vi "PH_ImageOperator.get COG.vi"(1 "Image":T1, 5 "error in (no error)":errorcluster) -> (16 "CoG-x":sgl, 17 "CoG-y":sgl, 19 "error out":errorcluster)   [LabVIEW 2014, in "PH_ImageOperator.lvlib"]
doc: "This VI calculates the center of gravity of the image."
uses:
  PH_ImageOperator.lvlib
  <vilib>/vision/Image Controls.llb/IMAQ Image.ctl
  <vilib>/vision/NI_Vision_Development_Module.lvlib
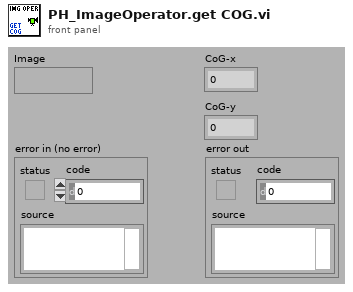
[diagram p1: front panel]
types:
  T1 = typedef "IMAQ Image.ctl" = refnum<image>
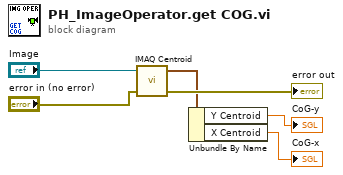
[diagram p0: block diagram]
diagram:
  n1 = call "IMAQ Centroid"("error in (no error)"="error in (no error)", "Image"="Image") -> ("error out"=→"error out":errorcluster, "Centroid"=w1:cluster{"X Centroid":sgl, "Y Centroid":sgl})  [unwired: 2 in]
  n2 = Unbundle By Name(w1) -> ("Y Centroid"=→"CoG-y":sgl, "X Centroid"=→"CoG-x":sgl)
